vi "MOCKBEAR_Getter.vi"(8 "error in (no error)":errorcluster, 11 "MOCKBEAR in":refnum<class "MOCKBEAR.lvclass">) -> (0 "error out":errorcluster, 3 "MOCKBEAR Params":T1)   [LabVIEW 2021, in "MOCKBEAR.lvclass"]
uses:
  MOCKBEAR.lvclass
  MOCKBEAR.lvclass/MOCKBEAR.ctl
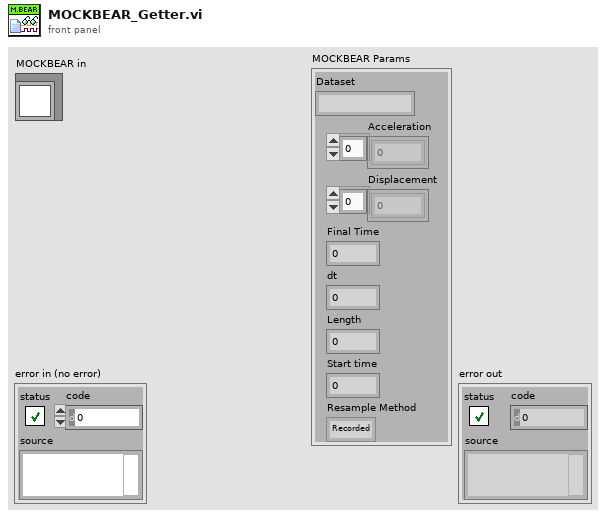
[diagram p1: front panel]
types:
  T1 = cluster{"Dataset":string, "Acceleration":dbl[], "Displacement":dbl[], "Final Time":dbl, "dt":dbl, "Length":i32, "Start time":i32, "Resample Method":enum16{"Recorded", "Auto Resample", "Custom Resample"}}
  T2 = enum16{"Recorded", "Auto Resample", "Custom Resample"}
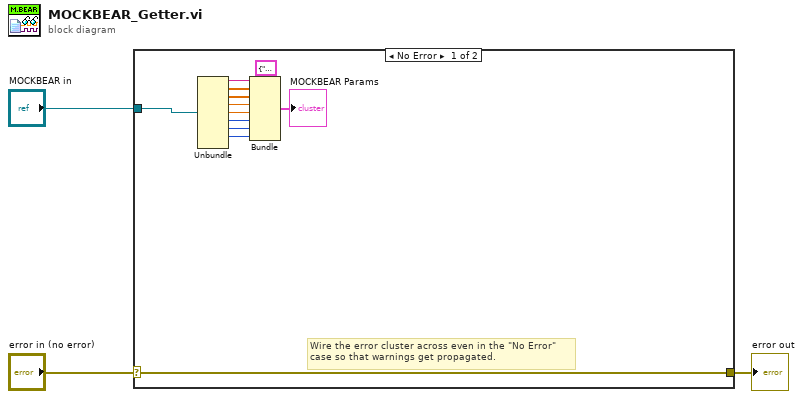
[diagram p0: block diagram]
diagram:
  n1 = case shown="No Error" "error in (no error)" {
    selector: "error in (no error)" -> [w15 w16]
    tunnel: [w15 w16] -> w2
    tunnel: "MOCKBEAR in" -> [w14 _]
    frame No Error {
      # "Wire the error cluster across even in the \"No Error\"\ncase so that warnings get propagated."
      n2 = Unbundle(w14) -> (w12:string, w11:dbl[], w10:dbl[], w9:dbl, w8:dbl, w7:i32, w6:u32, w5:T2)  [unwired: 1 out]
      n3 = Bundle(cluster=T1 {"Dataset"="", "Acceleration"=[], "Displacement"=[], "Final Time"=0.0, "dt"=0.0, "Length"=0, "Start time"=0, "Resample Method"=enum."Recorded"} ("Cluster of class private data"), "Dataset"=w12, "Acceleration"=w11, "Displacement"=w10, "Final Time"=w9, "dt"=w8, "Length"=w7, "Start time"=w6, "Resample Method"=w5) -> (→"MOCKBEAR Params":T1)
    }
    frame Error {
    }
  }
  "error out" <- w2
